vi "单线性扭转曲线图.vi"(2 "数组－数值 2":dbl[](array[numeric]), 3 "数组－数值":dbl[](array[numeric])) -> (0 "扭转刚度值":dbl, 1 "XY Graph":cluster{"Y":dbl[], "Y":dbl[]}[](graph) caption="弯曲刚度")   [LabVIEW 2016]
uses:
  <vilib>/Analysis/NI_AALPro.lvlib
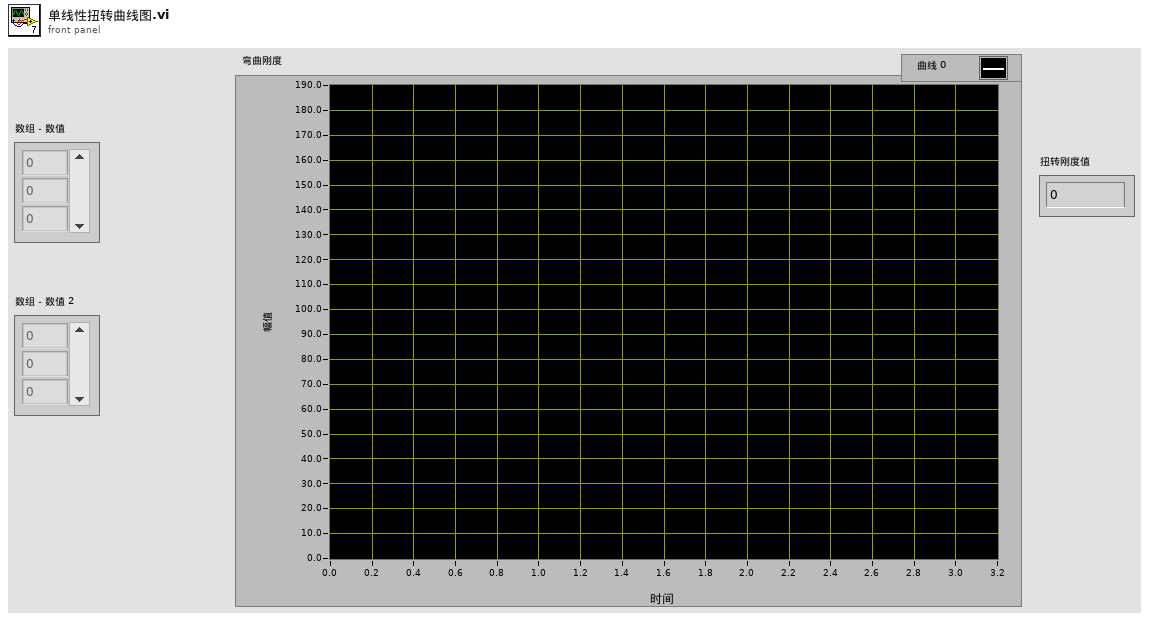
[diagram p1: front panel]
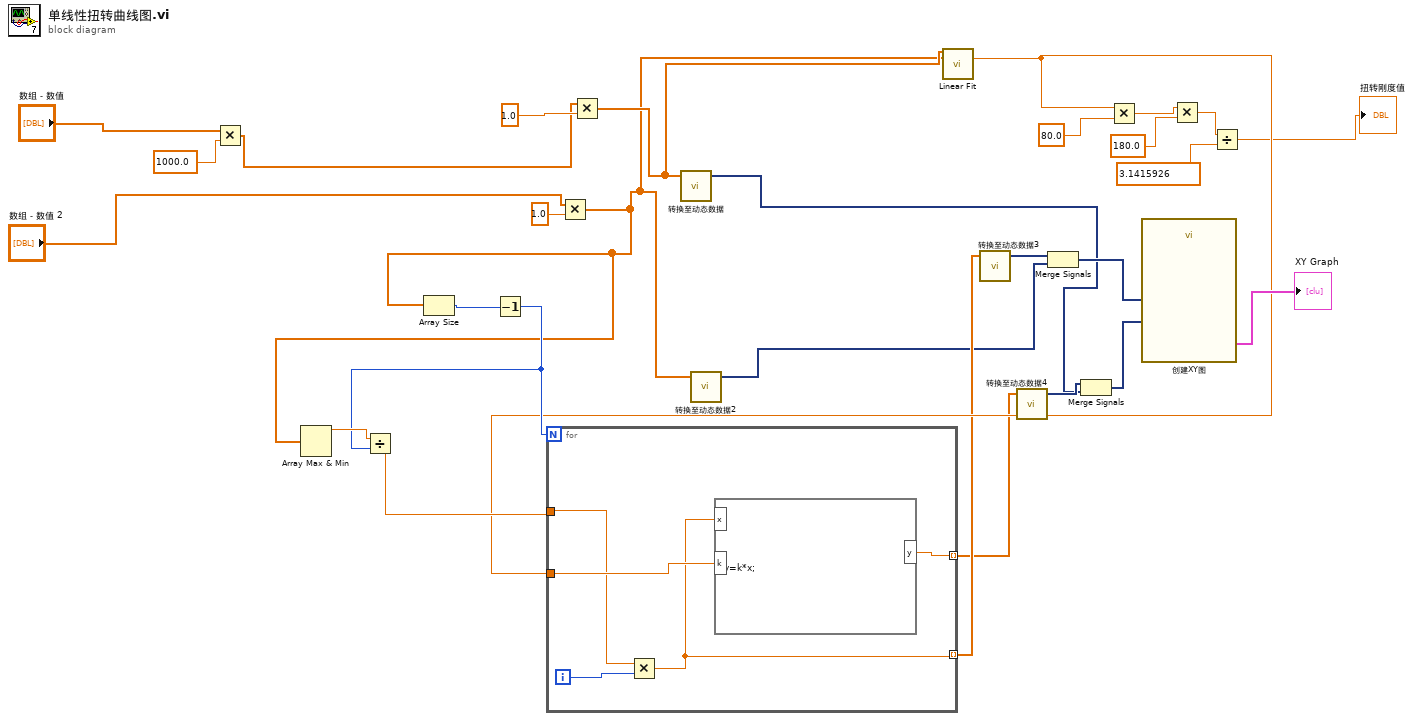
[diagram p0: block diagram]
diagram:
  n1 = Multiply(x="数组－数值", y=1000.0) -> (x*y=w15:dbl[])
  n2 = Multiply(x="数组－数值 2", y=1.0) -> (x*y=w7:dbl[])
  n3 = Array Max & Min(array=w7) -> (max value=w26:dbl)  [unwired: 3 out]
  n4 = Array Size(array=w7) -> (size(s)=w27:i32)
  n5 = Decrement(x=w27) -> (x-1=w25:i32)
  n6 = Divide(x=w26, y=w25) -> (x/y=w24:dbl)
  n7 = Multiply(x=w15, y=1.0) -> (x*y=w8:dbl[])
  n8 = call "转换至动态数据"("Array"=w8) -> ("Dynamic Data Type"=w2:dynamicdata)  [unwired: 3 in]
  n9 = call "转换至动态数据2"("Array"=w7) -> ("Dynamic Data Type"=w5:dynamicdata)  [unwired: 3 in]
  n10 = call <vilib>:"Linear Fit.vi"("Y"=w8, "X"=w7) -> ("slope"=w20:dbl)  [unwired: 9 in, 4 out]
  n11 = for {
    N: w25 -> [_]
    tunnel: w20 -> [w33]
    tunnel: [w32] -> w18 mode=indexing
    tunnel: [w29] -> w19 mode=indexing
    tunnel: w24 -> [w31]
    i -> [w30]
    n12 = Multiply(x=w31, y=w30) -> (x*y=w29:dbl)
    n13 = formula code="y=k*x;"("x"=w29, "k"=w33) -> ("y"=w32:dbl)
  }
  n14 = call "转换至动态数据3"("Array"=w19) -> ("Dynamic Data Type"=w6:dynamicdata)  [unwired: 3 in]
  n15 = call "转换至动态数据4"("Array"=w18) -> ("Dynamic Data Type"=w3:dynamicdata)  [unwired: 3 in]
  n16 = Merge Signals(w6, w5) -> (w4:dynamicdata)
  n17 = Merge Signals(w3, w2) -> (w1:dynamicdata)
  n18 = Multiply(x=w20, y=80.0) -> (x*y=w13:dbl)
  n19 = call "创建XY图"("Y Input"=w1, "X Input"=w4) -> ("XY Graph"=→"XY Graph":cluster{"X":dbl[], "Y":dbl[]}[])  [unwired: 8 in, 1 out]
  n20 = Multiply(x=w13, y=180.0) -> (x*y=w11:dbl)
  n21 = Divide(x=w11, y=3.1415926) -> (x/y=→"扭转刚度值":dbl)
